vi "testNetworkCamera.vi"() -> ()   [LabVIEW 2009, in "run.lvlib"]
uses:
  testing/run.lvlib
  Tools/Filing/FileSystem/FileSystem.lvclass
  CameraNetworkController.lvclass
  Tools/Filing/FileNeologist/FileNeologist.lvclass
panel:
  in  "remote address":string="192.168.104.186"
  in  "camera":string="Pixelfly"
  in  "save":bool
  in  "Configure":bool
  out "running":bool
  in  "Number of Images to take":i32=-1
  in  "close":bool
  in  "stop":bool
  in  "start":bool
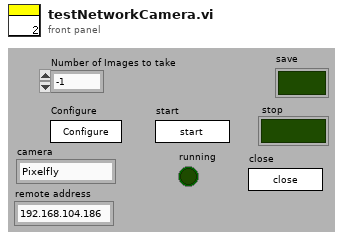
[diagram p1: front panel]
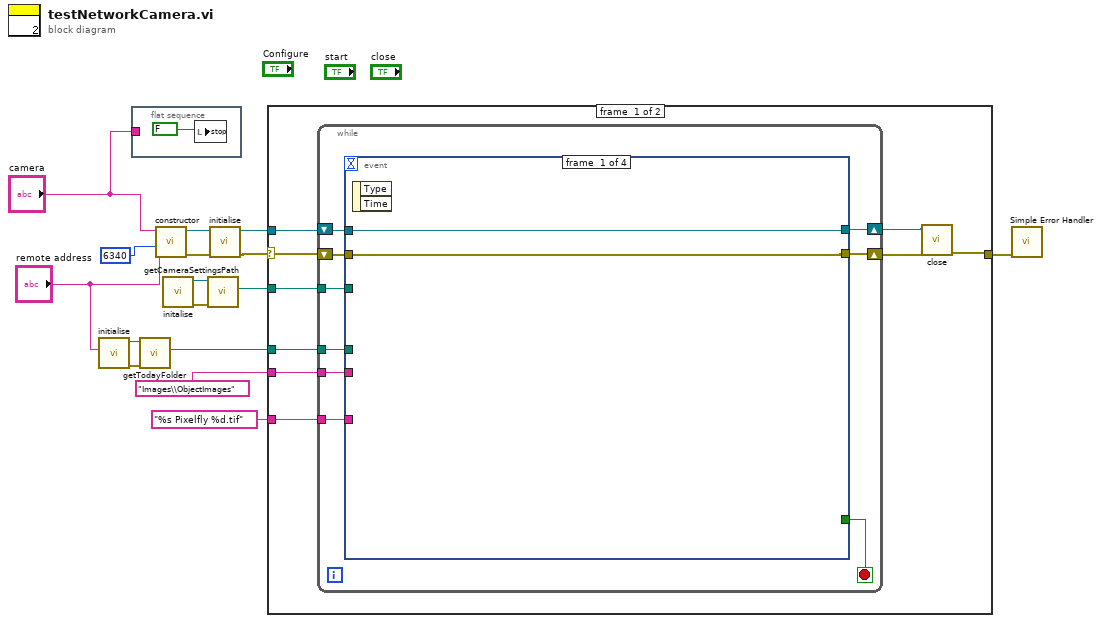
[diagram p0: block diagram]
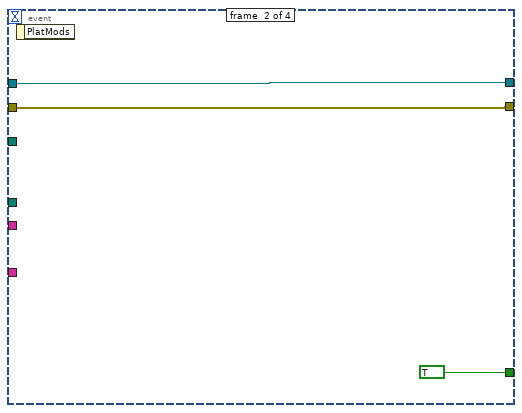
[diagram p2: hidden frame]
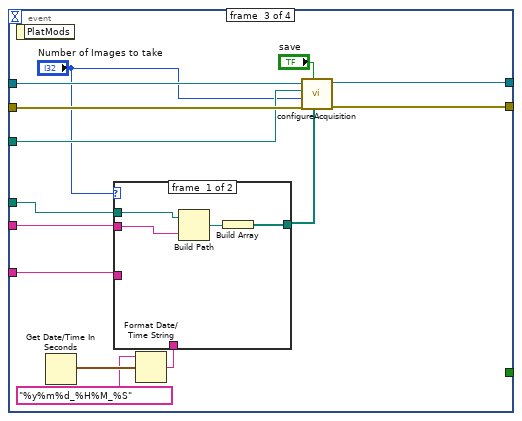
[diagram p3: hidden frame]
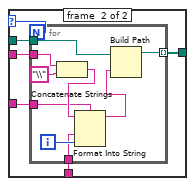
[diagram p4: hidden frame]
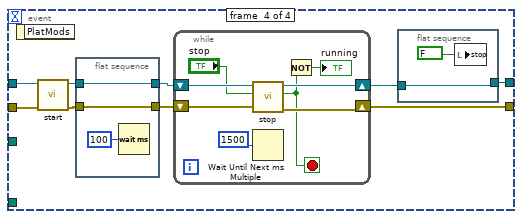
[diagram p5: hidden frame]
diagram:
  n1 = call "initialise.vi"("computer name"="remote address") -> ("error out"=w7:errorcluster, "FileNeologist out"=w8:refnum<class "FileNeologist.lvclass">)  [unwired: 9 in]
  n2 = flat-sequence {
    tunnel: "camera" -> [_]
    frame #0 {
      n3 = local write "stop"(FALSE) -> ()
    }
  }
  n4 = call "getTodayFolder.vi"("error in (no error)"=w7, "FileNeologist in"=w8) -> ("todayFolder"=w5:path)  [unwired: 7 in, 2 out]
  n5 = call "constructor.vi"("remote port"=u16 6340, "remote address"="remote address", "camera"="camera") -> ("error out"=w16:errorcluster, "CameraNetworkController out"=w15:refnum<class "CameraNetworkController.lvclass">)  [unwired: 7 in]
  n6 = call "initalise.vi"() -> ("error out"=w10:errorcluster, "FileSystem out"=w11:refnum<class "FileSystem.lvclass">)  [unwired: 10 in]
  n7 = call-dynamic "getCameraSettingsPath.vi"("error in (no error)"=w10, "FileSystem.lvclass in"=w11) -> ("CameraSettingsPath"=w9:path)  [unwired: 7 in, 2 out]
  n8 = call "initialise.vi"("error in (no error)"=w16, "CameraNetworkController in"=w15) -> ("error out"=w12:errorcluster, "CameraNetworkController out"=w14:refnum<class "CameraNetworkController.lvclass">)  [unwired: 8 in]
  n9 = case shown="No Error" w12 {
    selector: w12 -> [w25 w96]
    tunnel: w14 -> [w26 _]
    tunnel: w9 -> [w24 _]
    tunnel: w5 -> [w23 _]
    tunnel: "Images\\ObjectImages" -> [w22 _]
    tunnel: "%s Pixelfly %d.tif" -> [w21 _]
    tunnel: [w20 w96] -> w2
    frame #0 {
      n10 = while {
        tunnel: w24 -> [w32]
        tunnel: w23 -> [w31]
        tunnel: w22 -> [w30]
        tunnel: w21 -> [w29]
        shift-right: [w28] -> w18
        shift-left: w26 -> [w34]
        shift-right: [w27] -> w19
        shift-left: w25 -> [w33]
        stop <- w35 stop-if-true
        n11 = event shown="[3] \"start\": Mouse Down" {
          selector: _ -> [_ _ _ _]
          dyn-events: _ -> [_ _ _ _]
          timeout: _ -> [_ _ _ _]
          tunnel: [_ TRUE _ _] -> w35
          tunnel: w34 -> [w37 w38 w51 w82]
          tunnel: w33 -> [w36 w39 w50 w81]
          tunnel: w32 -> [_ _ w49 _]
          tunnel: w31 -> [_ _ w54 _]
          tunnel: w30 -> [_ _ w53 _]
          tunnel: w29 -> [_ _ w52 _]
          tunnel: [w37 w38 w46 w79] -> w28
          tunnel: [w36 w39 w45 w80] -> w27
          event #0 {
            n12 = event-data() -> ()  [unwired: 1 in, 2 out]
          }
          event #1 {
            n13 = event-data() -> ()  [unwired: 1 in, 1 out]
          }
          event #2 {
            n14 = event-data() -> ()  [unwired: 1 in, 1 out]
            n15 = Get Date/Time In Seconds() -> (seconds since 1Jan1904=w43:timestamp)
            n16 = Format Date/Time String(time format string (%c)="%y%m%d_%H%M_%S", seconds (now)=w43) -> (date/time string=w41:string)  [unwired: 1 in]
            n17 = case shown="1, Default" "Number of Images to take" {
              selector: "Number of Images to take" -> [_ w61]
              tunnel: w54 -> [w57 w64]
              tunnel: [w58 w63] -> w48
              tunnel: w52 -> [_ w62]
              tunnel: w53 -> [w56 w60]
              tunnel: w41 -> [_ w59]
              frame #0 {
                n18 = Build Path(base path=w57, name or relative path=w56) -> (appended path=w55:path)
                n19 = Build Array(w55) -> (w58:path[])
              }
              frame #1 {
                n20 = for {
                  N: w61 -> [_]
                  tunnel: w64 -> [w73]
                  tunnel: [w72] -> w63 mode=indexing
                  tunnel: w62 -> [w66]
                  tunnel: w60 -> [w71]
                  tunnel: w59 -> [w65]
                  i -> [w67]
                  n21 = Concatenate Strings(w71, "\\") -> (w68:string)
                  n22 = Format Into String(format string=w66, initial string=w68, w65, w67) -> (resulting string=w69:string)  [unwired: 1 in, 1 out]
                  n23 = Build Path(base path=w73, name or relative path=w69) -> (appended path=w72:path)
                }
              }
            }
            n24 = call "configureAcquisition.vi"("imagePaths"=w48, "save?"="save", "error in (no error)"=w50, "numberImages"="Number of Images to take", "settingsPath"=w49, "CameraNetworkController in"=w51) -> ("error out"=w45:errorcluster, "CameraNetworkController out"=w46:refnum<class "CameraNetworkController.lvclass">)  [unwired: 4 in]
          }
          event #3 {
            n25 = event-data() -> ()  [unwired: 1 in, 1 out]
            n26 = call "start.vi"("error in (no error)"=w81, "CameraNetworkController in"=w82) -> ("error out"=w76:errorcluster, "CameraNetworkController out"=w74:refnum<class "CameraNetworkController.lvclass">)  [unwired: 8 in]
            n27 = flat-sequence {
              tunnel: [w85] -> w77
              tunnel: w76 -> [w85]
              tunnel: [w83] -> w75
              tunnel: w74 -> [w83]
              frame #0 {
                n28 = Wait (ms)(milliseconds to wait=u32 100) -> ()  [unwired: 1 out]
              }
            }
            n29 = while {
              shift-right: [w94] -> w78
              shift-left: w75 -> [w95]
              shift-right: [w93] -> w80
              shift-left: w77 -> [w92]
              stop <- w90 stop-if-true
              n30 = call "stop.vi"("error in (no error)"=w92, "stop"="stop", "CameraNetworkController in"=w95) -> ("error out"=w93:errorcluster, "stopped?"=w90:bool, "CameraNetworkController out"=w94:refnum<class "CameraNetworkController.lvclass">)  [unwired: 6 in]
              n31 = Wait Until Next ms Multiple(millisecond multiple=1500) -> ()  [unwired: 1 out]
              n32 = Not(x=w90) -> (.not. x?=→"running":bool)
            }
            n33 = flat-sequence {
              tunnel: [w86] -> w79
              tunnel: w78 -> [w86]
              frame #0 {
                n34 = local write "stop"(FALSE) -> ()
              }
            }
          }
        }
      }
      n35 = call "close.vi"("error in (no error)"=w19, "CameraNetworkController in"=w18) -> ("error out"=w20:errorcluster)  [unwired: 8 in, 1 out]
    }
    frame #1 {
    }
  }
  n36 = call <vilib>:"Simple Error Handler.vi"("error in (no error)"=w2) -> ()  [unwired: 4 in, 5 out]
